vi "Stop Core.vi"(10 "final error code":i32, 11 "Controller in":refnum<class "Controller.lvclass">) -> (3 "Controller out":refnum<class "Controller.lvclass">)   [LabVIEW 2016, in "Controller Actor.lvlib" / "Controller.lvclass"]
uses:
  <userlib>/Common Components/Controller/Controller.lvclass
  <userlib>/Power-Requests-master/Power Availabilty Requests/Type Defs/Power Request Type.ctl
  <userlib>/Power-Requests-master/Power Availabilty Requests/Type Defs/Power Availiability Requests Functions.ctl
  <userlib>/Common Components/Controller/Controller.lvclass/Controller.ctl
  <vilib>/ActorFramework/Message Enqueuer/Message Enqueuer.lvclass/Message Enqueuer.ctl
  <vilib>/ActorFramework/Message Enqueuer/Enqueue.vi
  <vilib>/ActorFramework/Stop Msg/Stop Msg.lvclass
  C:/Program Files (x86)/National Instruments/LabVIEW 2016/vi.lib/ActorFramework/Message/Message.lvclass
  <vilib>/ActorFramework/Message Priority Queue/Priority Enqueue.vi
  <vilib>/ActorFramework/Message Enqueuer/Message Enqueuer.lvclass
  <vilib>/ActorFramework/Actor/Actor.lvclass
  <userlib>/Power-Requests-master/Power Requests.lvlib
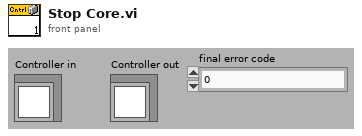
[diagram p1: front panel]
types:
  T1 = typedef "Power Requests.lvlib/Power Availiability Requests Functions.ctl" = enum32{"Power Create Request", "Power Set Request", "Power Clear Request", "Close Handle"}
  T2 = typedef "Power Requests.lvlib/Power Request Type.ctl" = enum32{"Power Request Display Required", "Power Request System Required", "Power Request Away Mode Required", "Power Request Execution Required"}
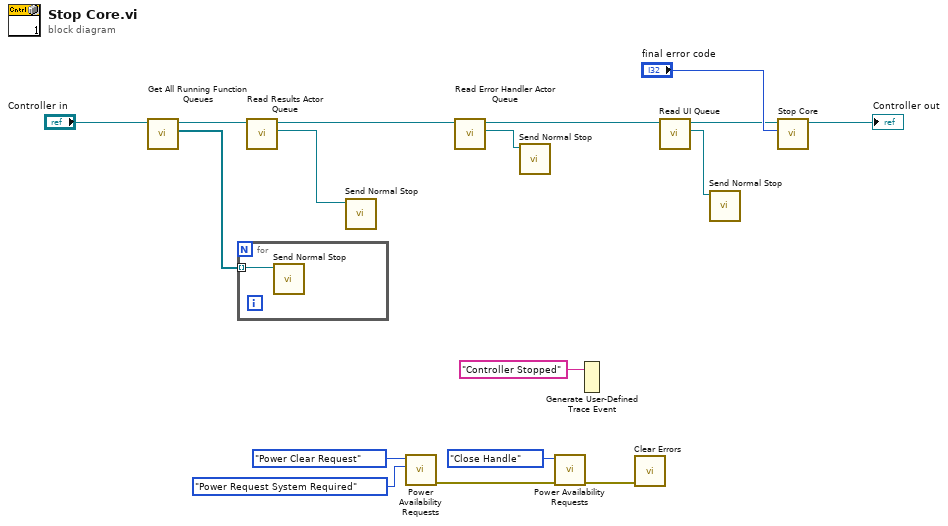
[diagram p0: block diagram]
diagram:
  n1 = call <userlib>:"Get All Running Function Queues.vi"("Controller in"="Controller in") -> ("Array of Function Queues"=w16:refnum<class "Message Enqueuer.lvclass">[], "Controller out"=w15:refnum<class "Controller.lvclass">)  [unwired: 8 in, 1 out]
  n2 = for {
    tunnel: w16 -> [w18] mode=indexing
    n3 = call <vilib>:"Send Normal Stop.vi"("Message Enqueuer"=w18) -> ()  [unwired: 10 in, 1 out]
  }
  n4 = call <userlib>:"Read Results Actor Queue.vi"("Controller in"=w15) -> ("Message Enqueuer"=w13:refnum<class "Message Enqueuer.lvclass">, "Controller out"=w11:refnum<class "Controller.lvclass">)  [unwired: 8 in, 1 out]
  n5 = call <vilib>:"Send Normal Stop.vi"("Message Enqueuer"=w13) -> ()  [unwired: 10 in, 1 out]
  n6 = call <userlib>:"Power Availability Requests.vi"("Power Request Type"=Power_Request_Type."Power Request System Required", "Power Availability Requests Functions"=Power_Availiability_Requests_Functions."Power Clear Request") -> ("error out"=w4:errorcluster)  [unwired: 8 in, 1 out]
  n7 = call <userlib>:"Read Error Handler Actor Queue.vi"("Controller in"=w11) -> ("Actor Framework.lvlib:Message Enqueuer"=w10:refnum<class "Message Enqueuer.lvclass">, "Controller out"=w8:refnum<class "Controller.lvclass">)  [unwired: 8 in, 1 out]
  n8 = call <vilib>:"Send Normal Stop.vi"("Message Enqueuer"=w10) -> ()  [unwired: 10 in, 1 out]
  n9 = call <userlib>:"Power Availability Requests.vi"("error in (no error)"=w4, "Power Availability Requests Functions"=Power_Availiability_Requests_Functions."Close Handle") -> ("error out"=w1:errorcluster)  [unwired: 8 in, 1 out]
  n10 = Generate User-Defined Trace Event(2:"Controller Stopped" ("trace string")) -> ()  [unwired: 1 in]
  n11 = call <vilib>:"Clear Errors.vi"("error in (no error)"=w1) -> ()  [unwired: 5 in, 2 out]
  n12 = call <userlib>:"Read UI Queue.vi"("UI Controller in"=w8) -> ("UI Queue"=w6:refnum<class "Message Enqueuer.lvclass">, "UI Controller out"=w7:refnum<class "Controller.lvclass">)  [unwired: 8 in, 1 out]
  n13 = call <vilib>:"Send Normal Stop.vi"("Message Enqueuer"=w6) -> ()  [unwired: 10 in, 1 out]
  n14 = call-parent "Stop Core.vi"("final error code"="final error code", "Actor in"=w7) -> ("Actor out"=→"Controller out":refnum<class "Controller.lvclass">)  [unwired: 9 in]
